vi "Test Subvi.vi"(10 "Boolean":bool, 11 "Array in":dbl[][](array[numeric])) -> (2 "Array out":dbl[][](array[numeric]), 3 "Waveform Chart":dbl[][](graph))   [LabVIEW 2024]
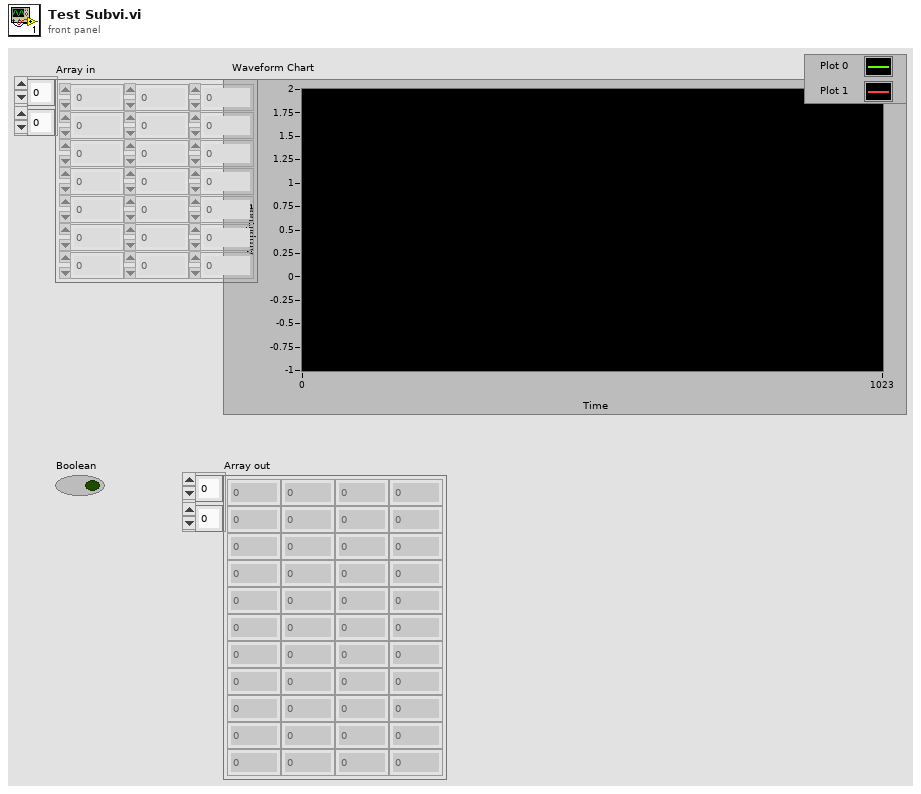
[diagram p1: front panel]
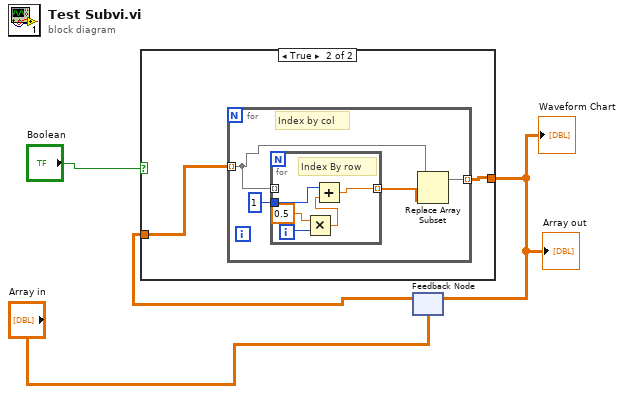
[diagram p0: block diagram]
diagram:
  n1 = feedback #1("Array in") -> (w3:dbl[][])
  n2 = case shown="True" "Boolean" {
    tunnel: [w5 w7] -> w2
    tunnel: w3 -> [w5 w6]
    frame False {
    }
    frame True {
      n3 = for {
        tunnel: w6 -> [w11] mode=indexing
        tunnel: [w9] -> w7 mode=indexing
        # "Index by col"
        n4 = for {
          tunnel: w11 -> [_] mode=indexing
          tunnel: [w16] -> w10 mode=indexing
          tunnel: 1 -> [w12]
          i -> [w13]
          # "Index By row"
          n5 = Multiply(x=0.5 ("element"), y=w13) -> (x*y=w15:dbl)
          n6 = Add(x=w12, y=w15) -> (x+y=w16:dbl)
        }
        n7 = Replace Array Subset(array=w11, new element=w10) -> (w9:dbl[])  [unwired: 1 in]
      }
    }
  }
  "Waveform Chart" <- w2
  "Array out" <- w2
  n8 = feedback-in #1(w2) -> ()
